vi "InitState.vi"(9 "Container State":T2, 11 "Control State in":T1) -> (3 "Control State out":T1)   [LabVIEW 2019, in "ExpandHorizontal.xctl"]
uses:
  ExpandHorizontal.xctl
  <vilib>/_xctls/Container State.ctl
  State.ctl
  <vilib>/_xctls/XControlSupport.lvlib
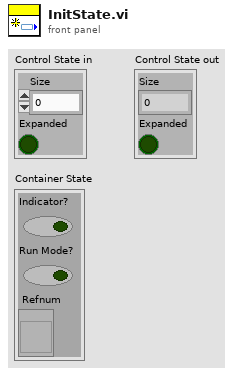
[diagram p1: front panel]
types:
  T1 = typedef "ExpandHorizontal.xctl/State.ctl" = cluster{"Size":i16, "Expanded":bool}
  T2 = typedef "XControlSupport.lvlib/Container State.ctl" = cluster{"Indicator?":bool, "Run Mode?":bool, " Refnum":refnum<vi>}
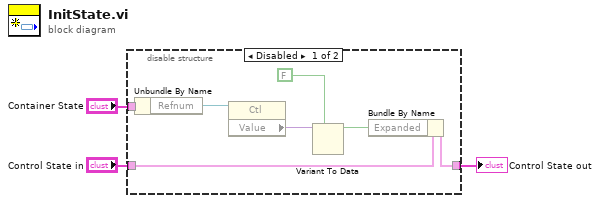
[diagram p0: block diagram]
diagram:
  n1 = disable-structure shown="Disabled" {
    disable-tunnel: "Container State" -> [w10 _]
    disable-tunnel: "Control State in" -> [w9 w11]
    disable-tunnel: [w5 w11] -> w1
    frame Disabled {
      n2 = Unbundle By Name(w10) -> ("Refnum"=w8:refnum<vi>)
      n3 = property class="Ctl"(reference=w8) -> ("Value"=w7:variant)  [unwired: 1 in, 2 out]
      n4 = Variant To Data(type=FALSE, Variant=w7) -> (data=w4:bool)  [unwired: 1 in, 1 out]
      n5 = Bundle By Name(cluster=w9, "Expanded"=w4) -> (w5:T1)
    }
    frame Enabled {
    }
  }
  "Control State out" <- w1
